vi "Dialog (Blacken).vi"(8 "error in (no error)":errorcluster, 9 "Transparency (40)":u8=40, 11 "Dialog in":refnum<class "Dialog.lvclass">) -> (0 "error out":errorcluster, 1 "timed out?":bool, 2 "Selection":string, 3 "Dialog out":refnum<class "Dialog.lvclass">)   [LabVIEW 2012, in "Dialog.lvlib" / "Dialog.lvclass"]
doc: "This VI wraps the Dialog Box VI and takes care of blackening the screen to keep the user focused on the dialog box.\nIf the Dialog Box VI is overriden, this VI will cast dynamically to the correct instance. There is no need to override this VI for blackening the screen in other dialog classes."
uses:
  Dialog.lvclass
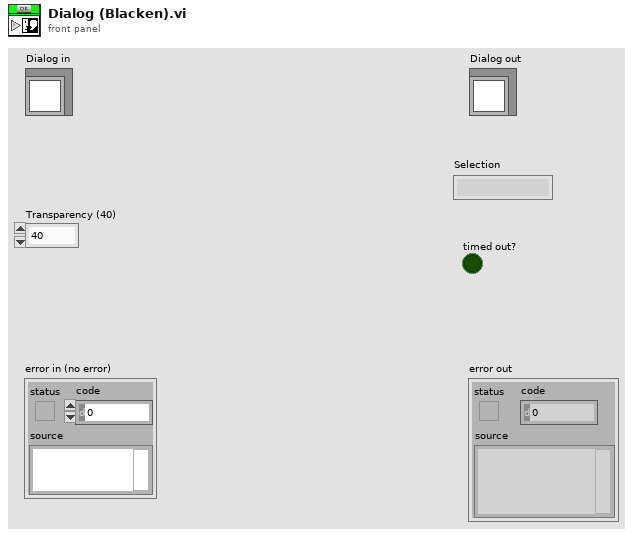
[diagram p1: front panel]
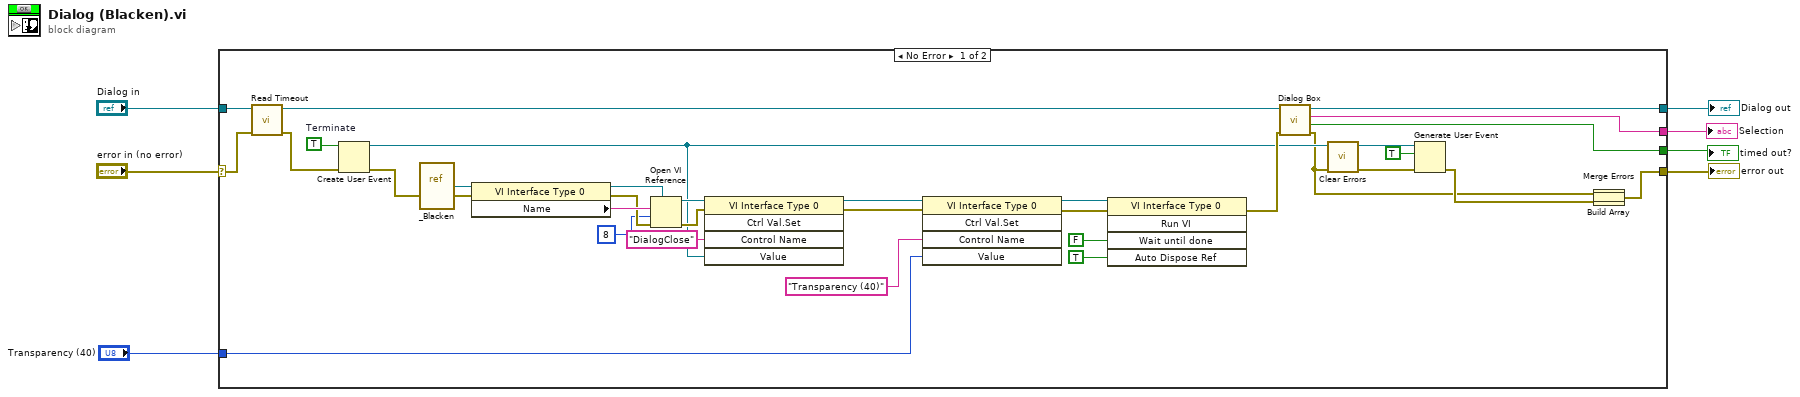
[diagram p0: block diagram]
diagram:
  n1 = case shown="No Error" "error in (no error)" {
    selector: "error in (no error)" -> [w18 w42]
    tunnel: [w33 w42] -> w6
    tunnel: [w35 w41] -> w4
    tunnel: "Dialog in" -> [w19 w41]
    tunnel: "Transparency (40)" -> [w20 _]
    tunnel: [w12 _] -> w2
    tunnel: [w11 _] -> w1
    frame No Error {
      w40 = TRUE  # Terminate
      n2 = call-dynamic "Read Timeout.vi"("error in (no error)"=w18, "Dialog.lvclass in"=w19) -> ("error out"=w17:errorcluster, "Dialog.lvclass out"=w14:refnum<class "Dialog.lvclass">)  [unwired: 8 out]
      n3 = Create User Event(user event datatype=w40, error in=w17) -> (user event=w13:refnum<user-event>, error out=w37:errorcluster)
      n4 = vi-ref "_Blacken.vi"() -> (w39:refnum<vi>)
      n5 = property class="VI Interface Type 0"(reference=w39, error in=w37) -> (reference out=w31:refnum<vi>, error out=w36:errorcluster, "Name"=w38:string)
      n6 = Open VI Reference(type specifier VI Refnum (for type only)=w31, vi path=w38, options=8, error in (no error)=w36) -> (vi reference=w30:refnum<vi>, error out=w29:errorcluster)  [unwired: 2 out]
      n7 = invoke class="VI Interface Type 0" method="Ctrl Val.Set"(reference=w30, error in=w29, "Control Name"="DialogClose", "Value"=w13) -> (reference out=w16:refnum<vi>, error out=w15:errorcluster)  [unwired: 1 in, 3 out]
      n8 = invoke class="VI Interface Type 0" method="Ctrl Val.Set"(reference=w16, error in=w15, "Control Name"="Transparency (40)", "Value"=w20) -> (reference out=w23:refnum<vi>, error out=w22:errorcluster)  [unwired: 1 in, 3 out]
      n9 = invoke class="VI Interface Type 0" method="Run VI"(reference=w23, error in=w22, "Wait until done"=FALSE ("Wait Until Done"), "Auto Dispose Ref"=TRUE ("Auto Dispose Reference")) -> (error out=w25:errorcluster)  [unwired: 1 in, 4 out]
      n10 = call-dynamic "Dialog Box.vi"("error in (no error)"=w25, "Dialog in"=w14) -> ("error out"=w8:errorcluster, "timed out?"=w12:bool, "Selection"=w11:string, "Dialog out"=w35:refnum<class "Dialog.lvclass">)  [unwired: 6 out]
      n11 = call <vilib>:"Clear Errors.vi"("error in (no error)"=w8) -> ("error out"=w9:errorcluster)  [unwired: 6 out]
      n12 = Generate User Event(user event=w13, event data cluster=TRUE ("event data"), error in=w9) -> (error out=w24:errorcluster)  [unwired: 1 out]
      n13 = Build Array(w8, w24) -> (w10:errorcluster[])
      n14 = Merge Errors(w10) -> (w33:errorcluster)
    }
    frame Error {
    }
  }
  "error out" <- w6
  "Dialog out" <- w4
  "timed out?" <- w2
  "Selection" <- w1
